vi "Pre Launch Init.vi"(11 "Nested in":refnum<class "Linear Encoder.lvclass">) -> (0 "error out":errorcluster, 3 "Nested out":refnum<class "Linear Encoder.lvclass">)   [LabVIEW 2020, in "Linear Encoder.lvlib" / "Linear Encoder.lvclass"]
doc: "(<B>Filename</B>: Actor Framework.lvlib:Actor.lvclass:Pre Launch Init.vi)\n\nDefines behavior that occurs after the Launch Nested Actor method is invoked but before the actor's Actor Core method begins running.\n\nBy default, this method does nothing. A descendant class may override it to define behavior."
uses:
  Linear Encoder.lvclass
  Linear Encoder.lvclass/Linear Encoder.ctl
  <vilib>/ActorFramework/Actor/Actor.lvclass
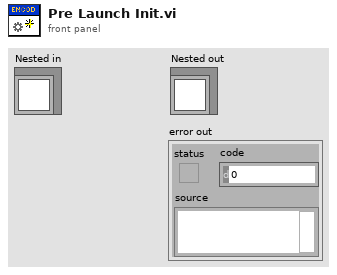
[diagram p1: front panel]
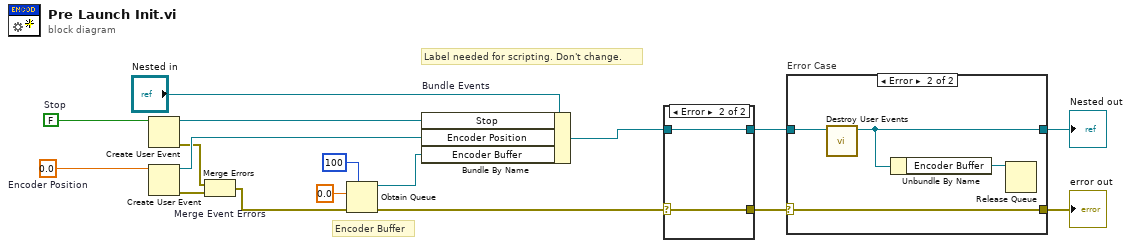
[diagram p0: block diagram]
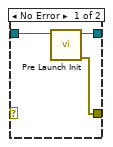
[diagram p2: hidden frame]
diagram:
  w9 = 0.0  # Encoder Position
  w16 = FALSE  # Stop
  # "Encoder Buffer"
  # "Label needed for scripting. Don't change."
  n1 = Create User Event(user event datatype=w16) -> (user event=w14:refnum<user-event>, error out=w4:errorcluster)  [unwired: 1 in]
  n2 = Create User Event(user event datatype=w9) -> (user event=w8:refnum<user-event>, error out=w7:errorcluster)  [unwired: 1 in]
  n3 = Merge Errors "Merge Event Errors"(w4, w7) -> (w3:errorcluster)
  n4 = Obtain Queue(max queue size (-1, unlimited)=100, element data type=0.0, error in (no error)=w3) -> (queue out=w5:refnum<queue>, error out=w2:errorcluster)  [unwired: 2 in, 1 out]
  n5 = Bundle By Name "Bundle Events"(cluster="Nested in", "Stop"=w14, "Encoder Position"=w8, "Encoder Buffer"=w5) -> (w11:refnum<class "Linear Encoder.lvclass">)
  n6 = case shown="Error" w2 {
    selector: w2 -> [_ w22]
    tunnel: [w20 w21] -> w12
    tunnel: w11 -> [w19 w21]
    tunnel: [w18 w22] -> w10
    frame No Error {
      n7 = call-parent "Pre Launch Init.vi"("Actor in"=w19) -> ("error out"=w18:errorcluster, "Actor out"=w20:refnum<class "Linear Encoder.lvclass">)  [unwired: 9 in]
    }
    frame Error {
    }
  }
  n8 = case "Error Case" shown="Error" w10 {
    selector: w10 -> [w23 w28]
    tunnel: w12 -> [w24 w27]
    tunnel: [w24 w26] -> w15
    tunnel: [w23 w28] -> w13
    frame No Error {
    }
    frame Error {
      n9 = call "Destroy User Events.vi"("UI Template in"=w27) -> ("UI Template out"=w26:refnum<class "Linear Encoder.lvclass">)  [unwired: 10 in]
      n10 = Unbundle By Name(w26) -> ("Encoder Buffer"=w25:refnum<queue>)
      n11 = Release Queue(queue=w25) -> ()  [unwired: 2 in, 3 out]
    }
  }
  "error out" <- w13
  "Nested out" <- w15
